vi "Get AIM Hardware Parameters.vi"(8 "error in":errorcluster, 11 "custom device":T5=18446744073709551615 format="%.0x") -> (0 "error out":errorcluster, 2 "aim hardware parameters":T1, 3 "custom device out":T5 format="%.0x")   [LabVIEW 2020, in "AIM MIL-STD-1553 Scripting.lvlib"]
doc: "Returns <b>aim hardware parameters</b> such as PXI Slot Number and BIU Number as configured in the specified <b>custom device</b>. This VI does not perform device discovery."
uses:
  AIM MIL-STD-1553 Scripting.lvlib
  <vilib>/NI VeriStand/Custom Device API/Custom Device Item Ref.ctl
  Shared/AIM Hardware Parameters.ctl
  Shared/Initialization Method.ctl
  Shared/Bus Selection.ctl
  Shared/Coupling Mode.ctl
  Constants.vi
  <vilib>/NI VeriStand/Custom Device API/Get Item Property (U16).vi
  <vilib>/NI VeriStand/Custom Device API/Get Item Property (I32).vi
  <vilib>/NI VeriStand/Custom Device API/Custom Device API.lvlib
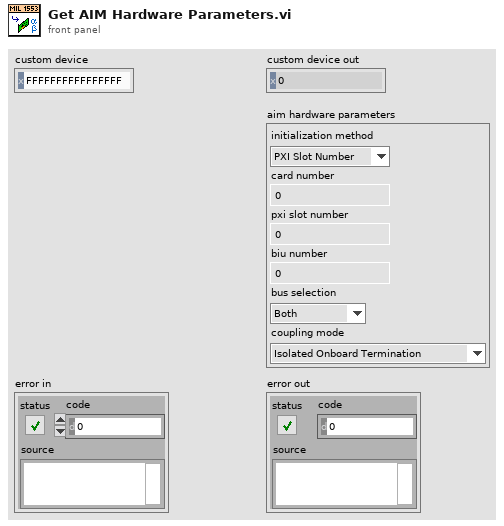
[diagram p1: front panel]
types:
  T1 = typedef "AIM Hardware Parameters.ctl" = cluster{"initialization method":T2, "card number":i32, "pxi slot number":i32, "biu number":i32, "bus selection":T3, "coupling mode":T4}
  T2 = typedef "Initialization Method.ctl" = enum16{"PXI Slot Number", "Card Number"}
  T3 = typedef "Bus Selection.ctl" = enum16{"Both", "Primary", "Secondary"}
  T4 = typedef "Coupling Mode.ctl" = enum16{"Isolated Onboard Termination", "Transformer Coupled", "Direct Coupled", "External with Onboard Termination", "Onboard Digital Wrap-around"}
  T5 = typedef "Custom Device API.lvlib/Custom Device Item Ref.ctl" = u64
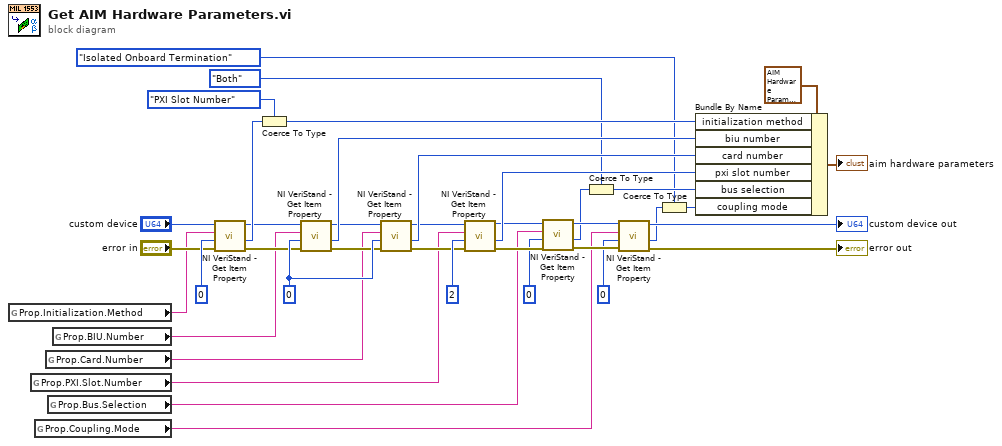
[diagram p0: block diagram]
diagram:
  w38 = 0 ("Default Value")
  n1 = global read "Constants.vi" "Prop.Initialization.Method"() -> (w23:string)
  n2 = global read "Constants.vi" "Prop.PXI.Slot.Number"() -> (w20:string)
  n3 = global read "Constants.vi" "Prop.Coupling.Mode"() -> (w9:string)
  n4 = global read "Constants.vi" "Prop.Card.Number"() -> (w21:string)
  n5 = global read "Constants.vi" "Prop.Bus.Selection"() -> (w10:string)
  n6 = global read "Constants.vi" "Prop.BIU.Number"() -> (w22:string)
  n7 = call-poly <vilib>:"NI VeriStand - Get Item Property.vi"("error in (no error)"="error in", "Default Value"=u16 0, "Property Name"=w23, "Item Ref in"="custom device") -> ("error out"=w26:errorcluster, "Value"=w33:u16, "Item Ref out"=w25:T5)  [unwired: 4 in, 1 out]
  n8 = Coerce To Type(0:w33, 1:Initialization_Method."PXI Slot Number" ("initialization method")) -> (2:w24:T2)
  n9 = call-poly <vilib>:"NI VeriStand - Get Item Property.vi"("error in (no error)"=w26, "Default Value"=w38, "Property Name"=w22, "Item Ref in"=w25) -> ("error out"=w31:errorcluster, "Value"=w36:i32, "Item Ref out"=w32:T5)  [unwired: 4 in, 1 out]
  n10 = call-poly <vilib>:"NI VeriStand - Get Item Property.vi"("error in (no error)"=w31, "Default Value"=w38, "Property Name"=w21, "Item Ref in"=w32) -> ("error out"=w29:errorcluster, "Value"=w35:i32, "Item Ref out"=w30:T5)  [unwired: 4 in, 1 out]
  n11 = call-poly <vilib>:"NI VeriStand - Get Item Property.vi"("error in (no error)"=w29, "Default Value"=2, "Property Name"=w20, "Item Ref in"=w30) -> ("error out"=w16:errorcluster, "Value"=w34:i32, "Item Ref out"=w15:T5)  [unwired: 4 in, 1 out]
  n12 = call-poly <vilib>:"NI VeriStand - Get Item Property.vi"("error in (no error)"=w16, "Default Value"=u16 0, "Property Name"=w10, "Item Ref in"=w15) -> ("error out"=w13:errorcluster, "Value"=w3:u16, "Item Ref out"=w14:T5)  [unwired: 4 in, 1 out]
  n13 = Coerce To Type(0:w3, 1:Bus_Selection."Both" ("bus selection")) -> (2:w4:T3)
  n14 = call-poly <vilib>:"NI VeriStand - Get Item Property.vi"("error in (no error)"=w13, "Default Value"=u16 0, "Property Name"=w9, "Item Ref in"=w14) -> ("error out"=→"error out":errorcluster, "Value"=w6:u16, "Item Ref out"=→"custom device out":T5)  [unwired: 4 in, 1 out]
  n15 = Coerce To Type(0:w6, 1:Coupling_Mode."Isolated Onboard Termination" ("coupling mode")) -> (2:w5:T4)
  n16 = Bundle By Name(cluster=T1 {"initialization method"=enum."PXI Slot Number", "card number"=0, "pxi slot number"=0, "biu number"=0, "bus selection"=enum."Both", "coupling mode"=enum."Isolated Onboard Termination"} ("device parameters"), "initialization method"=w24, "biu number"=w36, "card number"=w35, "pxi slot number"=w34, "bus selection"=w4, "coupling mode"=w5) -> (→"aim hardware parameters":T1)
